vi "Read configuration item.vi"(8 "error in (no error)":errorcluster, 10 "configuration item":string, 11 "IConfigDBQueries in":refnum<class "mysql-queries.lvclass">) -> (0 "error out":errorcluster, 2 "result":string)   [LabVIEW 2020, in "mysql-queries.lvlib" / "mysql-queries.lvclass"]
uses:
  mysql-queries.lvclass
  mysql-queries.lvclass/mysql-queries.ctl
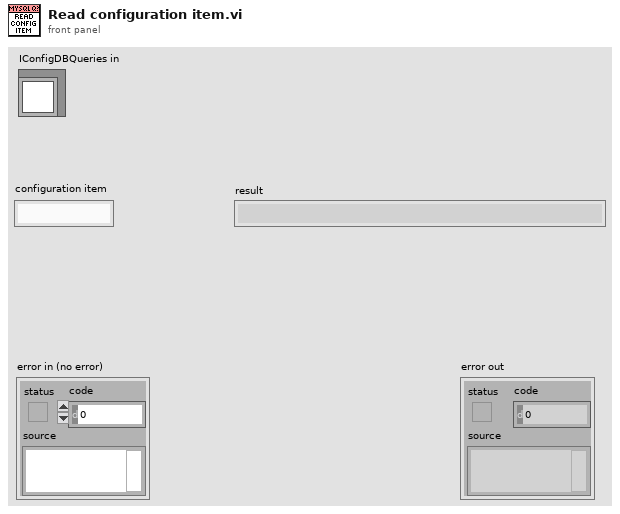
[diagram p1: front panel]
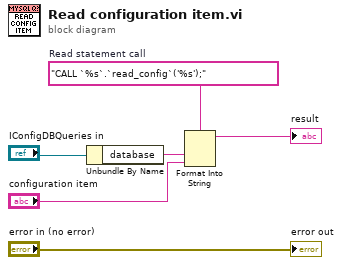
[diagram p0: block diagram]
diagram:
  w6 = "CALL `%s`.`read_config`('%s');"  # Read statement call
  n1 = Unbundle By Name("IConfigDBQueries in") -> ("database"=w4:string)
  n2 = Format Into String(format string=w6, w4, "configuration item") -> (resulting string=→"result":string)  [unwired: 2 in, 1 out]
  "error out" <- "error in (no error)"
